vi "Másodperc_átalakító.vi"(9 "Másodperc érték":i32, 10 "Perc érték":i32, 11 "Óra érték":i32) -> (2 "Az összes érték másodpercben":i32)   [LabVIEW 2014]
doc: "Ez a SubVI átváltja a bemenetén érkezõ órákat percre, ehhez hozzáadja a bemeneti perceket, ezt átváltja másodpercre, majd hozzáadja bemeneti másodperceket, így a kimeneti értéket már csak másodpercekben kapjuk meg."
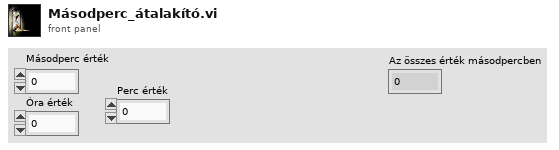
[diagram p1: front panel]
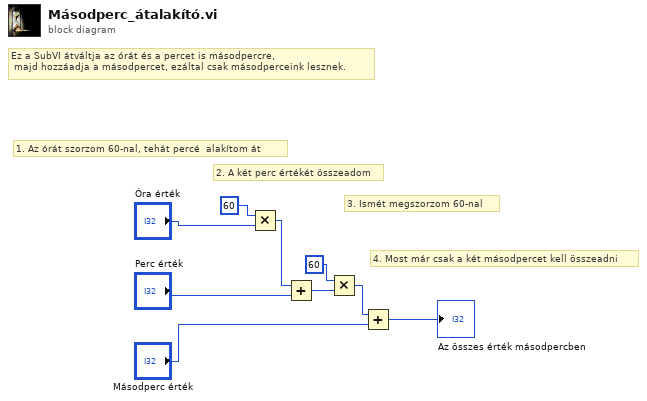
[diagram p0: block diagram]
diagram:
  # "4. Most már csak a két másodpercet kell összeadni"
  # "3. Ismét megszorzom 60-nal"
  # "2. A két perc értékét összeadom"
  # "1. Az órát szorzom 60-nal, tehát percé  alakítom át"
  # "Ez a SubVI átváltja az órát és a percet is másodpercre,\n majd hozzáadja a másodpercet, ezáltal csak másodperceink lesznek."
  n1 = Multiply(x=60 ("y"), y="Óra érték") -> (x*y=w6:i32)
  n2 = Add(x=w6, y="Perc érték") -> (x+y=w5:i32)
  n3 = Multiply(x=60, y=w5) -> (x*y=w7:i32)
  n4 = Add(x=w7, y="Másodperc érték") -> (x+y=→"Az összes érték másodpercben":i32)
